vi "Tosca-Execute MATLAB Script.vi"(0 "Path":string, 7 "Args":string, 9 "Fs":dbl, 11 "error in (no error)":errorcluster) -> (4 "result":string, 8 "output":string, 15 "error out":errorcluster)   [LabVIEW 2020]
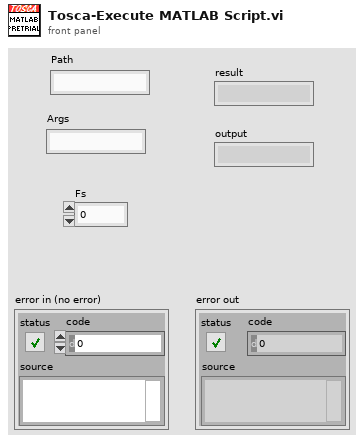
[diagram p1: front panel]
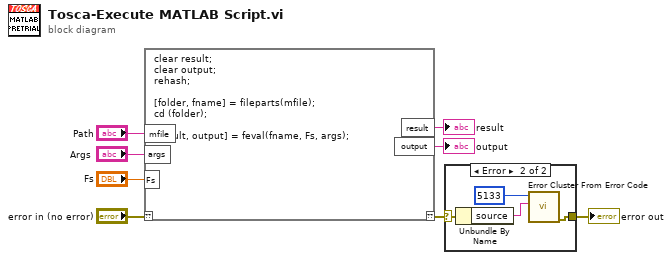
[diagram p0: block diagram]
diagram:
  n1 = script code="clear result;\nclear output;\nrehash;\n\n[folder, fname] = fileparts(mfile);\ncd (folder);\n\n[result, output] = feval(fname, Fs, args);"("??"="error in (no error)", "mfile"="Path", "args"="Args", "Fs"="Fs") -> ("??"=w3:errorcluster, "result"=→"result":string, "output"=→"output":string)
  n2 = case shown="Error" w3 {
    selector: w3 -> [w9 w11]
    tunnel: [w9 w12] -> w2
    frame No Error {
    }
    frame Error {
      n3 = Unbundle By Name(w11) -> ("source"=w10:string)
      n4 = call <vilib>:"Error Cluster From Error Code.vi"("error message (\"\")"=w10, "error code (0)"=5133) -> ("error out"=w12:errorcluster)  [unwired: 7 in]
    }
  }
  "error out" <- w2
